vi "Write Sequential Addresses.vi"(7 "Target IC (1-8)":u8, 8 "error in (no error)":errorcluster, 9 "Data":u16[](array[numeric]) format="%04x", 10 "Starting Address":u16 format="%04x", 11 "FPGA Interface in":refnum<class "FPGA Interface.lvclass">) -> (0 "error out":errorcluster)   [LabVIEW 2020, in "BCI-1553 API.lvlib" / "FPGA Interface.lvlib" / "FPGA Interface.lvclass"]
doc: "Writes values to a series of consecutive addresses on a component in the 1553 Session. Sequential addressing cannot be used on addresses from 0x0400 to 0x0800."
uses:
  FPGA Interface.lvclass
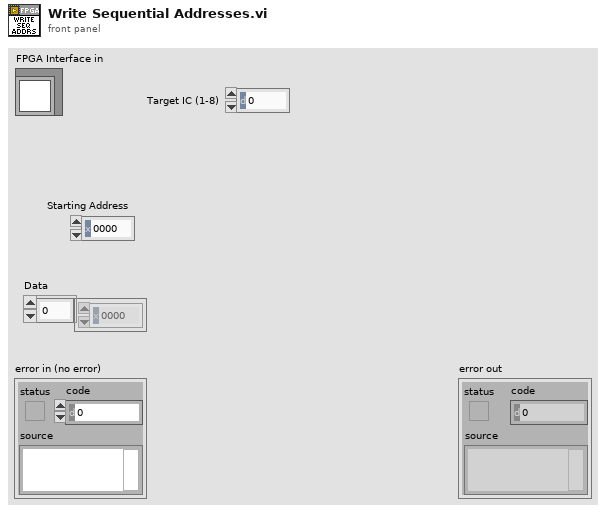
[diagram p1: front panel]
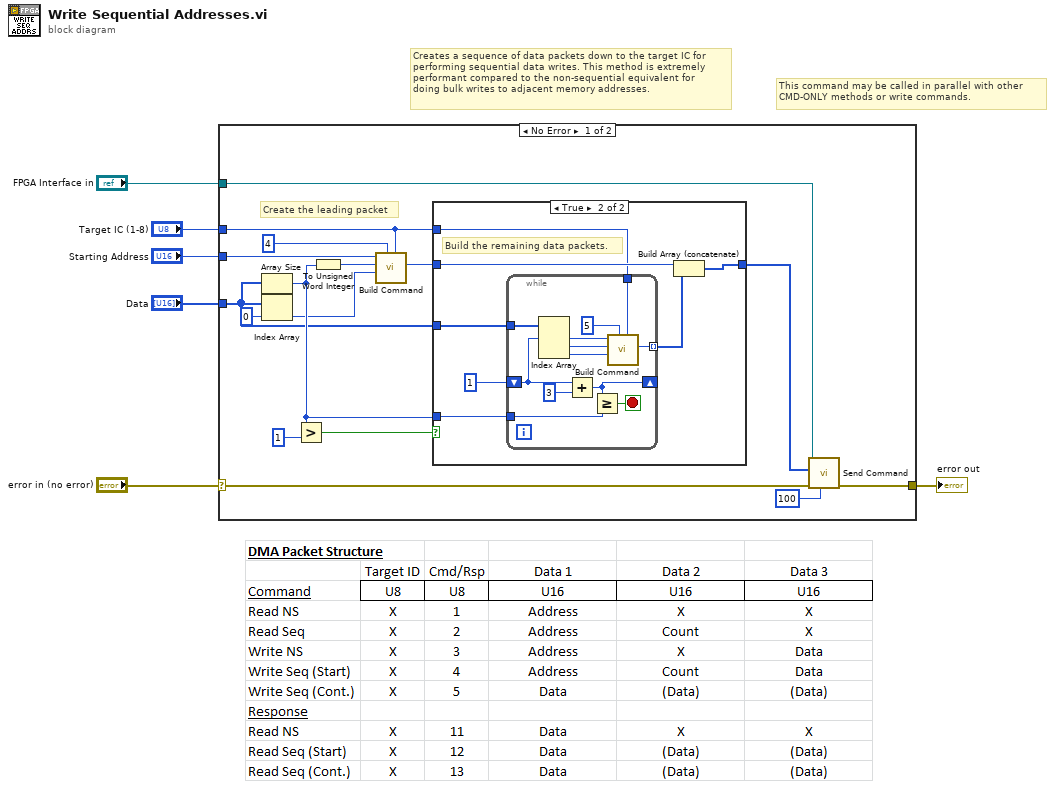
[diagram p0: block diagram]
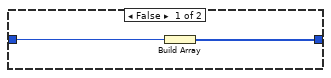
[diagram p2: hidden frame]
diagram:
  # "This command may be called in parallel with other\nCMD-ONLY methods or write commands."
  # "Creates a sequence of data packets down to the target IC for\nperforming sequential data writes. This method is extremely\nperformant compared to the non-sequential equivalent for\ndoing bulk writes to adjacent memory addresses."
  n1 = case shown="No Error" "error in (no error)" {
    selector: "error in (no error)" -> [w14 w44]
    tunnel: [w13 w44] -> w5
    tunnel: "FPGA Interface in" -> [w21 _]
    tunnel: "Target IC (1-8)" -> [w12 _]
    tunnel: "Starting Address" -> [w20 _]
    tunnel: "Data" -> [w11 _]
    frame No Error {
      # "Create the leading packet"
      n2 = Array Size(array=w11) -> (size(s)=w17:i32)
      n3 = Index Array(array=w11, index=0) -> (element=w10:u16)
      n4 = Greater?(x=w17, y=1) -> (0:w18:bool)
      n5 = To Unsigned Word Integer(number=w17) -> (unsigned 16bit integer=w9:u16)
      n6 = call "Build Command.vi"("Target"=w12, "CMD ID"=u8 4, "Data 3"=w10, "Data 2"=w9, "Data 1"=w20) -> ("Command"=w16:u64)  [unwired: 5 in, 1 out]
      n7 = case shown="True" w18 {
        tunnel: w11 -> [_ w29]
        tunnel: w17 -> [_ w25]
        tunnel: w16 -> [w24 w31]
        tunnel: [w23 w30] -> w15
        tunnel: w12 -> [_ w28]
        frame False {
          n8 = Build Array(w24) -> (w23:u64[])
        }
        frame True {
          # "Build the remaining data packets."
          n9 = while {
            tunnel: w29 -> [w43]
            tunnel: w28 -> [w38]
            tunnel: [w37] -> w27 mode=indexing
            shift-right: [w34] -> _
            shift-left: 1 -> [w36]
            tunnel: w25 -> [w33]
            stop <- w32 stop-if-true
            n10 = Index Array(array=w43, index #1=w36) -> (element #1=w42:u16, element #2=w41:u16, element #3=w40:u16)  [unwired: 2 in]
            n11 = Add(x=w36, y=3) -> (x+y=w34:i32)
            n12 = Greater Or Equal?(x=w34, y=w33) -> (x >= y?=w32:bool)
            n13 = call "Build Command.vi"("Target"=w38, "CMD ID"=u8 5, "Data 3"=w40, "Data 2"=w41, "Data 1"=w42) -> ("Command"=w37:u64)  [unwired: 5 in, 1 out]
          }
          n14 = Build Array (concatenate)(w31, w27) -> (w30:u64[])
        }
      }
      n15 = call "Send Command.vi"("Timeout (ms)"=100, "error in (no error)"=w14, "Data"=w15, "FPGA Interface in"=w21) -> ("error out"=w13:errorcluster)  [unwired: 7 in]
    }
    frame Error {
    }
  }
  "error out" <- w5
